vi "Develop Tools - ScratchPad.vi"() -> ()   [LabVIEW 2011]
uses:
  <vilib>/Utility/miscctls.llb/LVPositionTypeDef.ctl
panel:
  in  "Switched until released":T1 {"HSlide" scale=0.0..10.0; "VSlide" scale=0.0..10.0}
  in  "Switched when released":T1 {"HSlide" scale=0.0..10.0; "VSlide" scale=0.0..10.0}
  in  "Switched when pressed":T1 {"HSlide" scale=0.0..10.0; "VSlide" scale=0.0..10.0}
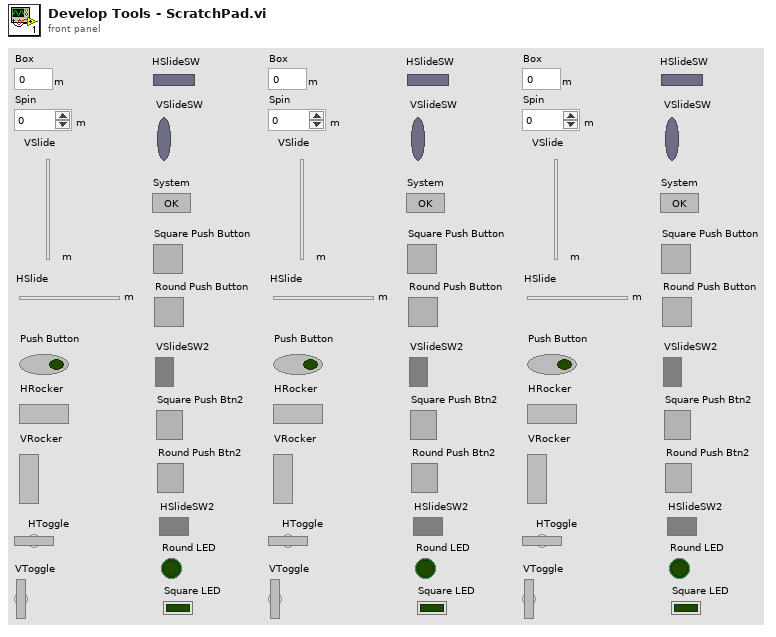
[diagram p1: front panel]
types:
  T1 = cluster{"Box":dbl[unit], "Spin":dbl[unit], "VSlide":dbl[unit], "HSlide":dbl[unit], "Push Button":bool, "HRocker":bool, "VRocker":bool, "HToggle":bool, "VToggle":bool, "HSlideSW":bool, "VSlideSW":bool, "System":bool, "Square Push Button":bool, "Round Push Button":bool, "VSlideSW2":bool, "Square Push Btn2":bool, "Round Push Btn2":bool, "HSlideSW2":bool, "Round LED":bool, "Square LED":bool}
  T2 = typedef "LVPositionTypeDef.ctl" = cluster{"Left":i32, "Top":i32}
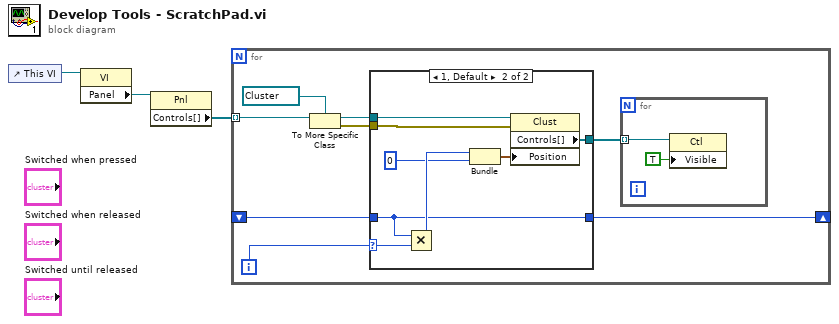
[diagram p0: block diagram]
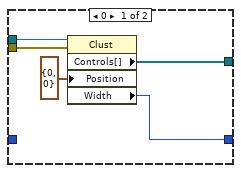
[diagram p2: hidden frame]
diagram:
  n1 = control-ref of="This VI"() -> (w3:refnum<vi>)
  n2 = property class="VI"(reference=w3) -> ("Panel"=w2:refnum<vi>)  [unwired: 1 in, 2 out]
  n3 = property class="Pnl"(reference=w2) -> ("Controls[]"=w1:refnum<vi>[])  [unwired: 1 in, 2 out]
  n4 = for {
    tunnel: w1 -> [w7] mode=indexing
    shift-right: [w5] -> _
    shift-left: _ -> [w4]
    i -> [w6]
    n5 = To More Specific Class(target class=refnum<vi> refnum ("reference"), reference=w7) -> (specific class reference=w10:refnum<vi>, error out=w8:errorcluster)  [unwired: 1 in]
    n6 = case shown="1, Default" w6 {
      selector: w6 -> [_ w17]
      tunnel: [w16 w22] -> w11
      tunnel: w10 -> [w15 w24]
      tunnel: w8 -> [w14 w23]
      tunnel: [w12 w18] -> w5
      tunnel: w4 -> [_ w18]
      frame 0 {
        n7 = property class="Clust"(reference=w15, error in=w14, "Position"=T2 {"Left"=0, "Top"=0}) -> ("Controls[]"=w16:refnum<vi>[], "Width"=w12:u32)  [unwired: 2 out]
      }
      frame 1, Default {
        n8 = Multiply(x=w18, y=w17) -> (x*y=w20:u32)
        n9 = Bundle(w20, 0) -> (w21:cluster{u32, i32})  [unwired: 1 in]
        n10 = property class="Clust"(reference=w24, error in=w23, "Position"=w21) -> ("Controls[]"=w22:refnum<vi>[])  [unwired: 2 out]
      }
    }
    n11 = for {
      tunnel: w11 -> [w26] mode=indexing
      n12 = property class="Ctl"(reference=w26, "Visible"=TRUE) -> ()  [unwired: 1 in, 2 out]
    }
  }
